vi "Disconnect.vi"(8 "error in":errorcluster, 11 "firebase in":refnum<class "firebase.lvclass">) -> (0 "error out":errorcluster)   [LabVIEW 2019, in "firebase.lvclass"]
uses:
  firebase.lvclass
  firebase.lvclass/firebase.ctl
  Get session.vi
  <vilib>/NI/Advanced HTTP Client/Session.lvclass
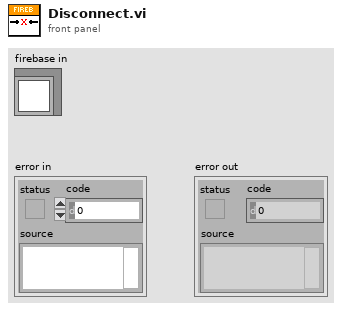
[diagram p1: front panel]
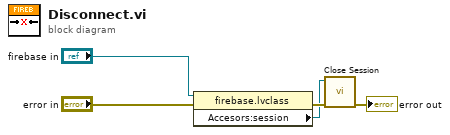
[diagram p0: block diagram]
diagram:
  n1 = property class="firebase.lvclass"(reference="firebase in", error in="error in") -> (error out=w4:errorcluster, "Accesors:session"=w1:refnum<class "Session.lvclass">)  [unwired: 1 out]
  n2 = call <vilib>:"Close Session.vi"("error in"=w4, "session"=w1) -> ("error out"=→"error out":errorcluster)  [unwired: 9 in]
